vi "P4CMD Dialog_HistHaveSymbol.vi"(6 "have revision":string, 10 "history info":string[][](array[string])) -> (2 "symbols":i32[](array[numeric]))   [LabVIEW 2020, in "NI_SCC_P4CMD.lvlib"]
uses:
  <vilib>/SourceControl/Providers/P4CMD/NI_SCC_P4CMD.lvlib
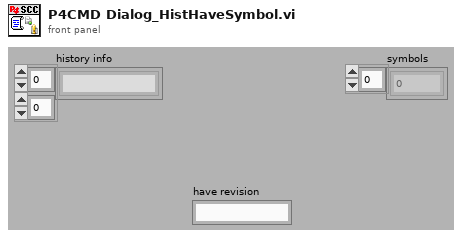
[diagram p1: front panel]
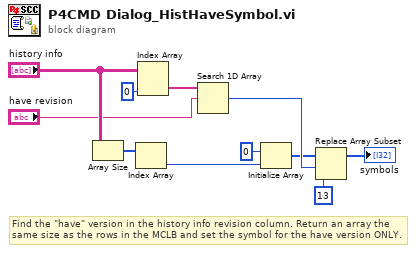
[diagram p0: block diagram]
diagram:
  # "Find the \"have\" version in the history info revision column. Return an array the same size as the rows in the MCLB and set the symbol for the have version ONLY."
  n1 = Array Size(array="history info") -> (size(s)=w4:i32[])
  n2 = Index Array(array=w4) -> (element=w3:i32)  [unwired: 1 in]
  n3 = Index Array(array="history info", index (col)=0 ("disabled index (col)")) -> (element=w6:string[])  [unwired: 1 in]
  n4 = Search 1D Array(1D array=w6, element="have revision") -> (index of element=w9:i32)  [unwired: 1 in]
  n5 = Initialize Array(0, w3) -> (w8:i32[])
  n6 = Replace Array Subset(array=w8, new element=13 ("new element/subarray"), index=w9) -> (→"symbols":i32[])
